vi "read 1b u8 number.vi"(8 "error in (no error)":errorcluster, 11 "TCP Network Connection in":refnum<k5>) -> (0 "error out":errorcluster, 2 "number":u8, 3 "TCP Network Connection out":refnum<k5>)   [LabVIEW 2020]
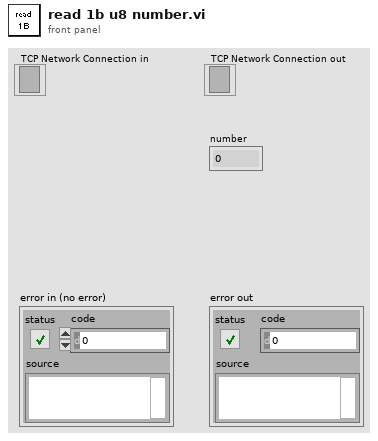
[diagram p1: front panel]
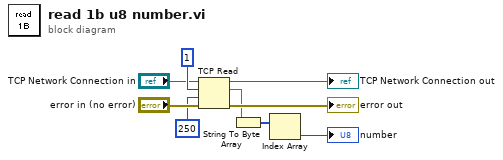
[diagram p0: block diagram]
diagram:
  n1 = TCP Read(connection ID="TCP Network Connection in", bytes to read=1, error in (no error)="error in (no error)", 9:250 ("timeout ms (25000)")) -> (connection ID out=→"TCP Network Connection out":refnum<k5>, data out=w6:string, error out=→"error out":errorcluster)  [unwired: 1 in]
  n2 = String To Byte Array(string=w6) -> (unsigned byte array=w7:u8[])
  n3 = Index Array(array=w7) -> (element=→"number":u8)  [unwired: 1 in]
